vi "currentScan.vi"(8 "error in (no error)":errorcluster, 10 "Imax":string, 11 "VISA resource name":refnum<visa-resource-name>) -> (0 "error out":errorcluster, 1 "max":bool, 2 "Istring":string, 3 "Ichart":dbl(graph))   [LabVIEW 2018]
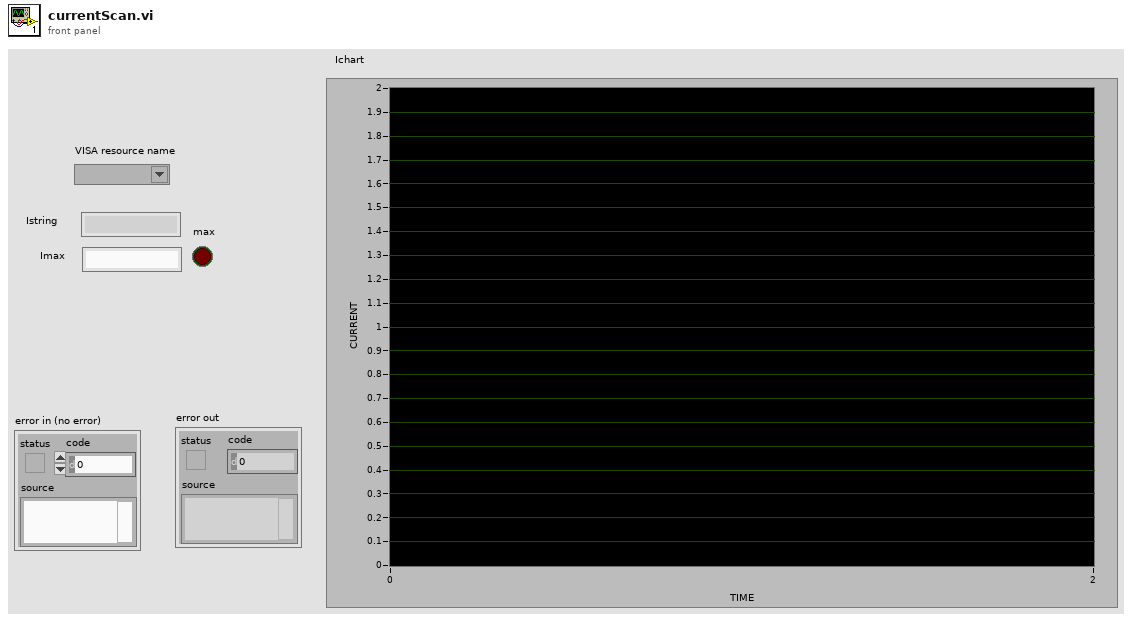
[diagram p1: front panel]
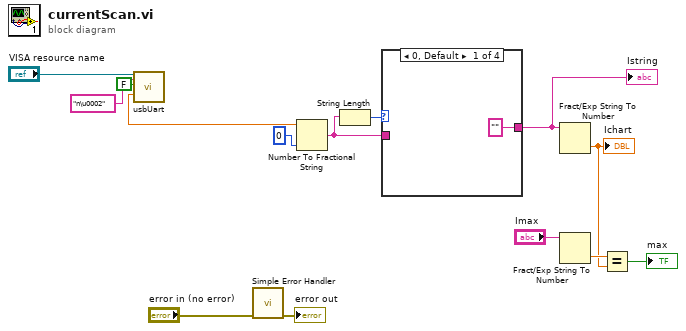
[diagram p0: block diagram]
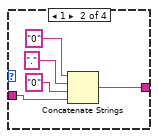
[diagram p2: hidden frame]
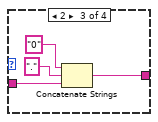
[diagram p3: hidden frame]
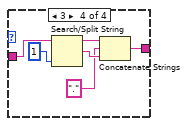
[diagram p4: hidden frame]
diagram:
  n1 = call "usbUart.vi"("VISA resource name"="VISA resource name", "write buffer"="n\u0002", "sdFeature"=FALSE) -> ("double precision float"=w7:dbl)  [unwired: 1 in, 15 out]
  n2 = call <vilib>:"Simple Error Handler.vi"("error in (no error)"="error in (no error)") -> ("error out"=→"error out":errorcluster)  [unwired: 4 in, 4 out]
  n3 = Number To Fractional String(number=w7, precision (6)=i16 0) -> (F-format string=w4:string)  [unwired: 2 in]
  n4 = String Length(string=w4) -> (length=w5:i32)
  n5 = case shown="0, Default" w5 {
    tunnel: w4 -> [_ w20 w21 w26]
    tunnel: ["" w16 w22 w25] -> w3
    frame 0, Default {
    }
    frame 1 {
      n6 = Concatenate Strings("0" ("string"), "." ("string"), "0" ("string"), w20) -> (w16:string)
    }
    frame 2 {
      n7 = Concatenate Strings("0" ("string"), "." ("string"), w21) -> (w22:string)
    }
    frame 3 {
      n8 = Search/Split String(string=w26, offset (0)=1) -> (substring before match=w29:string, match + rest of string=w28:string)  [unwired: 1 in, 1 out]
      n9 = Concatenate Strings(w29, "." ("string"), w28) -> (w25:string)
    }
  }
  "Istring" <- w3
  n10 = Fract/Exp String To Number(string=w3) -> (number=w2:dbl)  [unwired: 3 in, 1 out]
  "Ichart" <- w2
  n11 = Fract/Exp String To Number(string="Imax") -> (number=w11:dbl)  [unwired: 3 in, 1 out]
  n12 = Equal?(x=w11, y=w2) -> (x = y?=→"max":bool)
